vi "templates.vi"(7 "httpRequestID":u32) -> ()   [LabVIEW 2011]
doc: "This VI is a state machine that can be ran from a Browser."
uses:
  server/database/Users/User Record.ctl
  <vilib>/wsapi/NI_WebServices.lvlib
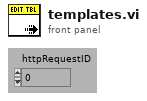
[diagram p1: front panel]
types:
  T1 = typedef "User Record.ctl" = cluster{"ixUser":i32, "sxUsername":string, "sLastName":string, "sFirstName":string, "sEmail":string, "sPassword":string, "tLoginTime":timestamp, "sLoginComputer":string, "fAdministrator":bool, "fRunSequences":bool, "fModifySequences":bool, "fRunScenarios":bool, "fModifyScenarios":bool, "fModifyTemplates":bool, "fModifyUsers":bool, "fModifyStations":bool, "fModifyFields":bool}
  T2 = typedef "Connection Refnum.ctl" = cluster{"Environment Handle":i32, "Connection Handle":i32}
  T3 = typedef "Keyed Array.ctl" = cluster{"keys":string[], "values":string[]}
  T4 = typedef "Template Record.ctl" = cluster{"ixTemplate":i32, "sxTemplateId":string, "sDescription":string, "sCreator":string, "tCreationDate":timestamp, "sModifier":string, "tModifiedDate":timestamp, "sType":string, "sStyle":string, "sFormat":string, "dWidth":dbl, "dHeight":dbl, "sFilename":string, "sScript":string, "sLayout":string, "sEditor":string, "sStyleProcess":string}
  T5 = cluster{"Local File Path":string, "Client File Name":string, "Content Type":string, "Size":u32}[]
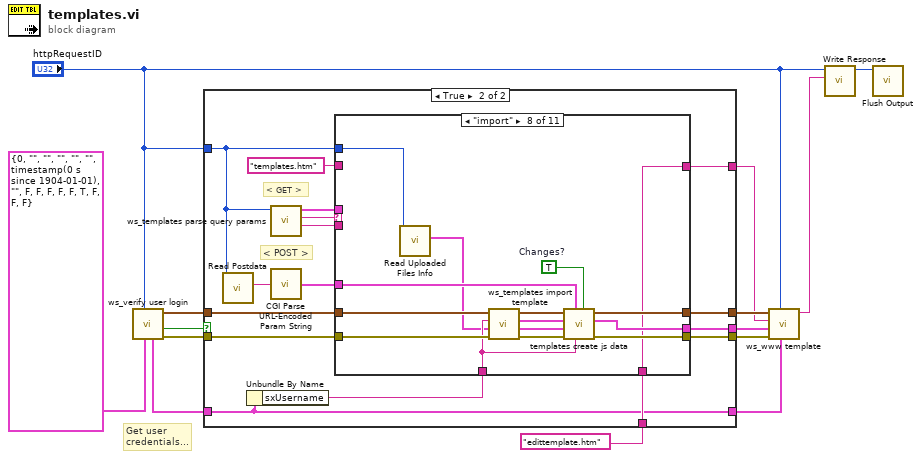
[diagram p0: block diagram]
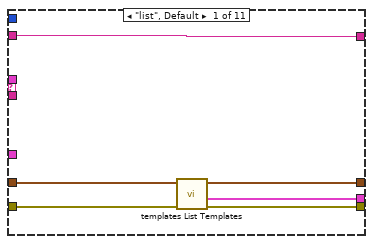
[diagram p3: hidden frame]
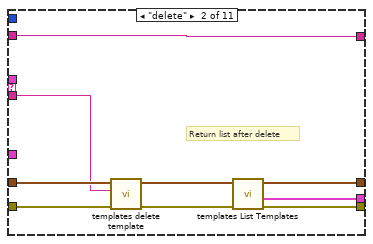
[diagram p4: hidden frame]
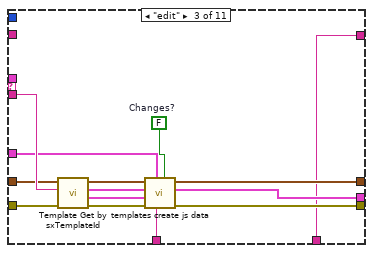
[diagram p5: hidden frame]
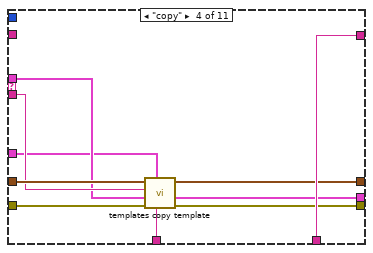
[diagram p6: hidden frame]
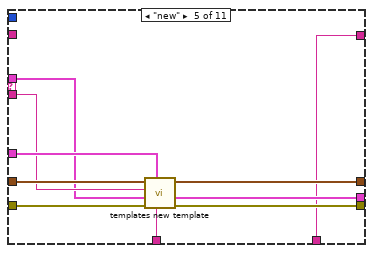
[diagram p7: hidden frame]
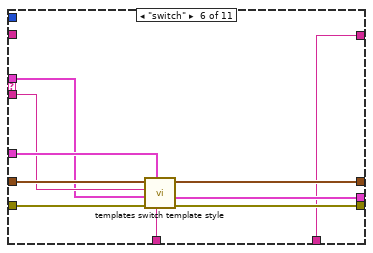
[diagram p8: hidden frame]
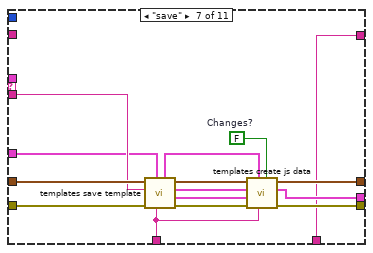
[diagram p9: hidden frame]
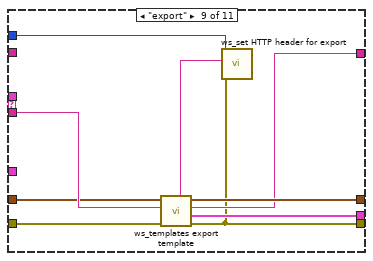
[diagram p10: hidden frame]
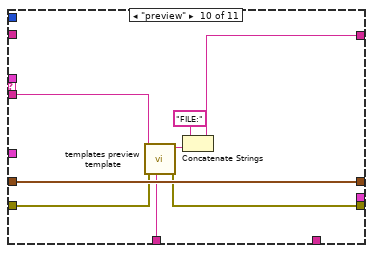
[diagram p11: hidden frame]
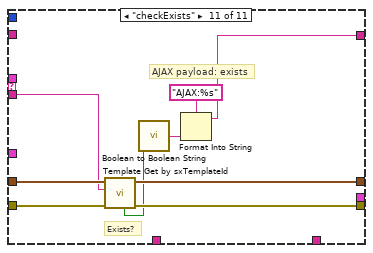
[diagram p12: hidden frame]
diagram:
  # "Get user \ncredentials..."
  n1 = call "ws_verify user login.vi"("Required Permisions"=T1 {"ixUser"=0, "sxUsername"="", "sLastName"="", "sFirstName"="", "sEmail"="", "sPassword"="", "tLoginTime"=timestamp(0 s since 1904-01-01), "sLoginComputer"="", "fAdministrator"=FALSE, "fRunSequences"=FALSE, "fModifySequences"=FALSE, "fRunScenarios"=FALSE, "fModifyScenarios"=FALSE, "fModifyTemplates"=TRUE, "fModifyUsers"=FALSE, "fModifyStations"=FALSE, "fModifyFields"=FALSE}, "httpRequestID"="httpRequestID") -> ("error out"=w6:errorcluster, "User Verified\nand Spartan\nAuthorized?"=w4:bool, "DB Connection Ref"=w5:T2, "User"=w3:T1)  [unwired: 6 in]
  n2 = case shown="True" w4 {
    tunnel: [w17 w25] -> w12
    tunnel: w3 -> [w15 w21]
    tunnel: w5 -> [w16 w26]
    tunnel: w6 -> [w17 w27]
    tunnel: "edittemplate.htm" ("Template (\"\")") -> [_ w29]
    tunnel: [w16 w24] -> w13
    tunnel: [_ w23] -> w10
    tunnel: [_ w22] -> w11
    tunnel: [w15 w21] -> w9
    tunnel: "httpRequestID" -> [_ w18]
    frame False {
    }
    frame True {
      # "< POST >"
      # "< GET >"
      n3 = call <vilib>:"Read Postdata.vi"("httpRequestID"=w18) -> ("postdata"=w19:string)  [unwired: 8 in, 2 out]
      n4 = Unbundle By Name(w21) -> ("sxUsername"=w28:string)
      n5 = call "ws_templates parse query params.vi"("httpRequestID"=w18) -> ("First Value"=w31:string, "First Key"=w20:string, "Query Parameters"=w30:T3)  [unwired: 8 in]
      n6 = call <vilib>:"CGI Parse URL-Encoded Param String.vi"("url-encoded param string"=w19) -> ("params"=w33:T3)
      n7 = case shown="\"import\"" w20 {
        tunnel: [w35 w46 w58 w65 w81 w91 w103 w118 w123 w135 w143] -> w25
        tunnel: w33 -> [_ _ w53 w67 w78 w88 w94 w116 _ _ _]
        tunnel: w27 -> [w36 w42 w60 w72 w82 w92 w97 w122 w130 w136 w146]
        tunnel: w26 -> [w38 w44 w61 w71 w79 w89 w96 w121 w129 w139 w145]
        tunnel: [w37 w47 w57 w64 w80 w90 w106 w117 w128 w139 w144] -> w24
        tunnel: "templates.htm" ("Template (\"\")") -> [w39 w48 _ _ _ _ _ _ _ _ _]
        tunnel: [w39 w48 w52 w68 w74 w84 w101 w113 w126 w137 w140] -> w23
        tunnel: [w34 w45 w54 w66 w75 w85 w105 w115 w127 _ _] -> w22
        tunnel: w31 -> [_ w40 w62 w70 w77 w87 w95 _ w131 w134 w142]
        tunnel: w30 -> [_ _ _ w69 w76 w86 _ _ _ _ _]
        tunnel: w28 -> [_ _ w49 w63 w73 w83 w98 w110 _ w132 _]
        tunnel: w29 -> [_ _ w52 w68 w74 w84 w101 w113 _ _ _]
        tunnel: w18 -> [_ _ _ _ _ _ _ w109 w125 _ _]
        frame "list", Default {
          n8 = call "templates List Templates.vi"("error in (no error)"=w36, "Connection Refnum In\n(0,0: Open New)"=w38) -> ("error out"=w35:errorcluster, "Template Keys"=w34:T3, "Connection Refnum In\n(0,0: Open New)"=w37:T2)  [unwired: 2 in, 5 out]
        }
        frame "delete" {
          # "Return list after delete"
          n9 = call "templates delete template.vi"("error in (no error)"=w42, "sxTemplateId (\"\")"=w40, "Connection Refnum In\n(0,0: Open New)"=w44) -> ("error out"=w41:errorcluster, "Connection Refnum In\n(0,0: Open New)"=w43:T2)  [unwired: 1 in, 6 out]
          n10 = call "templates List Templates.vi"("error in (no error)"=w41, "Connection Refnum In\n(0,0: Open New)"=w43) -> ("error out"=w46:errorcluster, "Template Keys"=w45:T3, "Connection Refnum In\n(0,0: Open New)"=w47:T2)  [unwired: 2 in, 5 out]
        }
        frame "edit" {
          w50 = FALSE  # Changes?
          n11 = call "Template Get by sxTemplateId.vi"("error in (no error)"=w60, "sxTemplateId (\"\")"=w62, "Connection Refnum"=w61) -> ("error out"=w59:errorcluster, "Parameters"=w51:T3, "Template Record"=w55:T4, "Connection Refnum"=w56:T2)  [unwired: 5 out]
          n12 = call "templates create js data.vi"("Changes?"=w50, "sxUsername"=w49, "POST Parameters"=w53, "error in (no error)"=w59, "template Parameters"=w51, "Template Record"=w55, "Connection Refnum"=w56) -> ("error out"=w58:errorcluster, "HTM Keys"=w54:T3, "Connection Refnum"=w57:T2)  [unwired: 2 out]
        }
        frame "copy" {
          n13 = call "templates copy template.vi"("username"=w63, "POST Parameters"=w67, "error in"=w72, "Keys in"=w69, "template"=w70, "Connection Refnum"=w71) -> ("error out"=w65:errorcluster, "Parameters"=w66:T3, "Connection Refnum"=w64:T2)  [unwired: 1 in, 2 out]
        }
        frame "new" {
          n14 = call "templates new template.vi"("user"=w73, "POST Parameters"=w78, "error in"=w82, "Keys in"=w76, "template STYLE"=w77, "Connection Refnum"=w79) -> ("error out"=w81:errorcluster, "HTM Keys out"=w75:T3, "Connection Refnum 2"=w80:T2)  [unwired: 3 out]
        }
        frame "switch" {
          n15 = call "templates switch template style.vi"("User"=w83, "POST Parameters"=w88, "error in (no error)"=w92, "Keys in"=w86, "sxTemplateId"=w87, "Connection Refnum In"=w89) -> ("error out"=w91:errorcluster, "HTM Keys out"=w85:T3, "Connection Refnum Out"=w90:T2)  [unwired: 3 out]
        }
        frame "save" {
          w99 = FALSE  # Changes?
          n16 = call "templates save template.vi"("sxUsername"=w98, "Post Parameters In"=w94, "error in (no error)"=w97, "sxTemplateId"=w95, "Connection Refnum"=w96) -> ("error out"=w107:errorcluster, "template parameters"=w100:T3, "New Template Record"=w102:T4, "Connection Refnum"=w104:T2, "Post Parameters Out"=w93:T3)  [unwired: 1 in, 1 out]
          n17 = call "templates create js data.vi"("Changes?"=w99, "sxUsername"=w98, "POST Parameters"=w93, "error in (no error)"=w107, "template Parameters"=w100, "Template Record"=w102, "Connection Refnum"=w104) -> ("error out"=w103:errorcluster, "HTM Keys"=w105:T3, "Connection Refnum"=w106:T2)  [unwired: 2 out]
        }
        frame "import" {
          w111 = TRUE  # Changes?
          n18 = call <vilib>:"Read Uploaded Files Info.vi"("httpRequestID"=w109) -> ("UploadedFilesList"=w108:T5)  [unwired: 8 in, 2 out]
          n19 = call "ws_templates import template.vi"("error in (no error)"=w122, "UploadedFilesList"=w108, "user"=w110, "Connection Refnum"=w121) -> ("error out"=w119:errorcluster, "template parameters"=w112:T3, "New Template Record"=w114:T4, "Connection Refnum"=w120:T2)  [unwired: 4 in]
          n20 = call "templates create js data.vi"("Changes?"=w111, "sxUsername"=w110, "POST Parameters"=w116, "error in (no error)"=w119, "template Parameters"=w112, "Template Record"=w114, "Connection Refnum"=w120) -> ("error out"=w118:errorcluster, "HTM Keys"=w115:T3, "Connection Refnum"=w117:T2)  [unwired: 2 out]
        }
        frame "export" {
          n21 = call "ws_templates export template.vi"("error out"=w130, "First Value"=w131, "Connection Refnum"=w129) -> ("error out 2"=w123:errorcluster, "empty keyed array"=w127:T3, "String"=w126:string, "Connection Refnum 2"=w128:T2, "Filename"=w124:string)  [unwired: 4 in]
          n22 = call "ws_set HTTP header for export.vi"("error in (no error)"=w123, "filename (\"\")"=w124, "httpRequestID"=w125) -> ()  [unwired: 8 in, 1 out]
        }
        frame "preview" {
          n23 = call "templates preview template.vi"("sxUsername"=w132, "error in (no error)"=w136, "sxTemplateID"=w134) -> ("error out"=w135:errorcluster, "PNG"=w133:string)  [unwired: 3 in, 4 out]
          n24 = Concatenate Strings("FILE:" ("format string"), w133) -> (w137:string)
        }
        frame "checkExists" {
          # "AJAX payload: exists"
          # "Exists?"
          n25 = call "Template Get by sxTemplateId.vi"("error in (no error)"=w146, "sxTemplateId (\"\")"=w142, "Connection Refnum"=w145) -> ("error out"=w143:errorcluster, "Connection Refnum"=w144:T2, "Data Present"=w141:bool)  [unwired: 6 out]
          n26 = call "Boolean to Boolean String.vi"("Boolean"=w141) -> ("Boolean string"=w148:string)  [unwired: 1 in]
          n27 = Format Into String(format string="AJAX:%s", w148) -> (resulting string=w140:string)  [unwired: 2 in, 1 out]
        }
      }
    }
  }
  n28 = call "ws_www template.vi"("User"=w9, "httpRequestID"="httpRequestID", "error in (no error)"=w12, "Template Keys (empty)"=w11, "Template (\"\")"=w10, "DB Connection Ref"=w13) -> ("HTTP Template Content"=w8:string)  [unwired: 5 in]
  n29 = call <vilib>:"Write Response.vi"("response string"=w8, "httpRequestID"="httpRequestID") -> ("httpRequestID out"=w7:u32)  [unwired: 8 in, 1 out]
  n30 = call <vilib>:"Flush Output.vi"("httpRequestID"=w7) -> ()  [unwired: 9 in, 2 out]
